vi "initialize client.vi"(8 "error in (no error)":errorcluster, 11 "Item Ref in":T1 format="%.0x") -> (0 "error out":errorcluster, 3 "Item Ref out":T1 format="%.0x")   [LabVIEW 2016]
uses:
  <vilib>/NI Veristand/Custom Device API/Custom Device Item Ref.ctl
  Shared/global constants.vi
  <vilib>/NI Veristand/Custom Device API/Set Item Property (Boolean).vi
  FPGA Resource Manager.lvlib
  <vilib>/NI VeriStand/Custom Device API/Custom Device API.lvlib
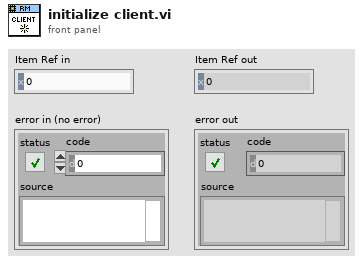
[diagram p1: front panel]
types:
  T1 = typedef "Custom Device API.lvlib/Custom Device Item Ref.ctl" = u64
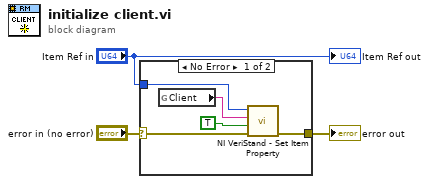
[diagram p0: block diagram]
diagram:
  n1 = case shown="No Error" "error in (no error)" {
    selector: "error in (no error)" -> [w5 w9]
    tunnel: [w4 w9] -> w2
    tunnel: "Item Ref in" -> [w8 _]
    frame No Error {
      n2 = global read "global constants.vi" "Client"() -> (w7:string)
      n3 = call-poly <vilib>:"NI VeriStand - Set Item Property.vi"("error in (no error)"=w5, "Value"=TRUE, "Property Name"=w7, "Item Ref in"=w8) -> ("error out"=w4:errorcluster)  [unwired: 5 in, 2 out]
    }
    frame Error {
    }
  }
  "error out" <- w2
  "Item Ref out" <- "Item Ref in"
